vi "VolumeScan.vi"() -> ()   [LabVIEW 2015]
panel:
  out "Image":T1(plugin-control)
  out "Status":string
  in  "Capture":bool
  in  "Tab Control":T2(tab)
  in  "Frames per position":u32
  in  "Camera settings":bool
  out "Status":bool
  out "Temperature":dbl
  in  "Camera identity":u16(ring) items=["Andor Ixon", "Dummy", "Manual", "PCO Edge", "PointGrey Grasshopper"]
  in  "Exposure (s)":dbl=0.1
  in  "Volume Wizard":bool
  in  "Imaging Locations":dbl[][](array[numeric])
  in  "XYZ Position":dbl[](array[numeric])
  in  "Save":T3(ring)
  in  "Path":path=path "G:/"
  in  "File Prefix":string="Map"
  in  "Stage VISA":refnum<visa-resource-name>="COM5"
  in  "remote controlled":bool
  in  "closed loop controlled":bool
  in  "VISA resource name":refnum<visa-resource-name>="COM4"
  in  "Shut Down":bool
  # "Piezo"
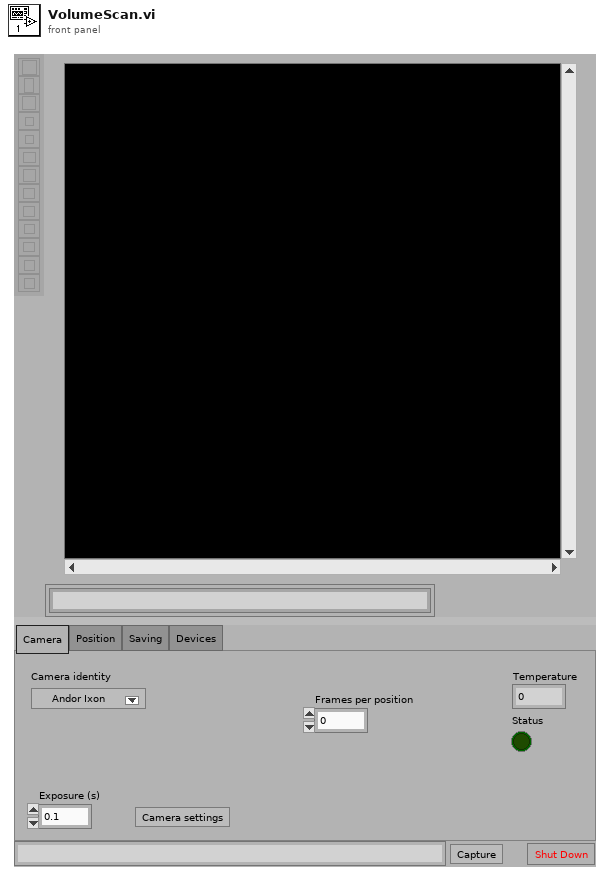
[diagram p1: front panel]
types:
  T1 = typedef "IMAQ Image.ctl" = refnum<image>
  T2 = enum32{"Camera", "Position", "Saving", "Devices"}
  T3 = enum16{"Don't save", "Save U16", "Save PNG", "Save TIFF"}
  T4 = enum16{"Initialize", "Shut down", "Set capture mode", "Set exposure", "Trigger and read", "Get status", "Other settings"}
  T5 = typedef "Image Type" = u32
  T6 = enum16{"Initialize", "Close", "Move Absolute", "Get Position", "Move Relative", "Set Acceleration", "Get Acceleration", "Set Speed", "Get Speed", "Limit Switch Status", "Motor Status", "Stop (controlled)", "Stop (instant)"}
  T7 = enum16{"Initialize", "Close", "Set position", "Get position", "Closed loop on", "Closed loop off", "Remote control on", "Remote control off"}
  T8 = cluster{"System OK?":bool, "Current exposure":dbl, "Temperature":dbl, "ROI":cluster{"X":u32, "X2":u32, "Y":u32, "Y2":u32}, "Binning":cluster{"X":u32, "Y":u32}}
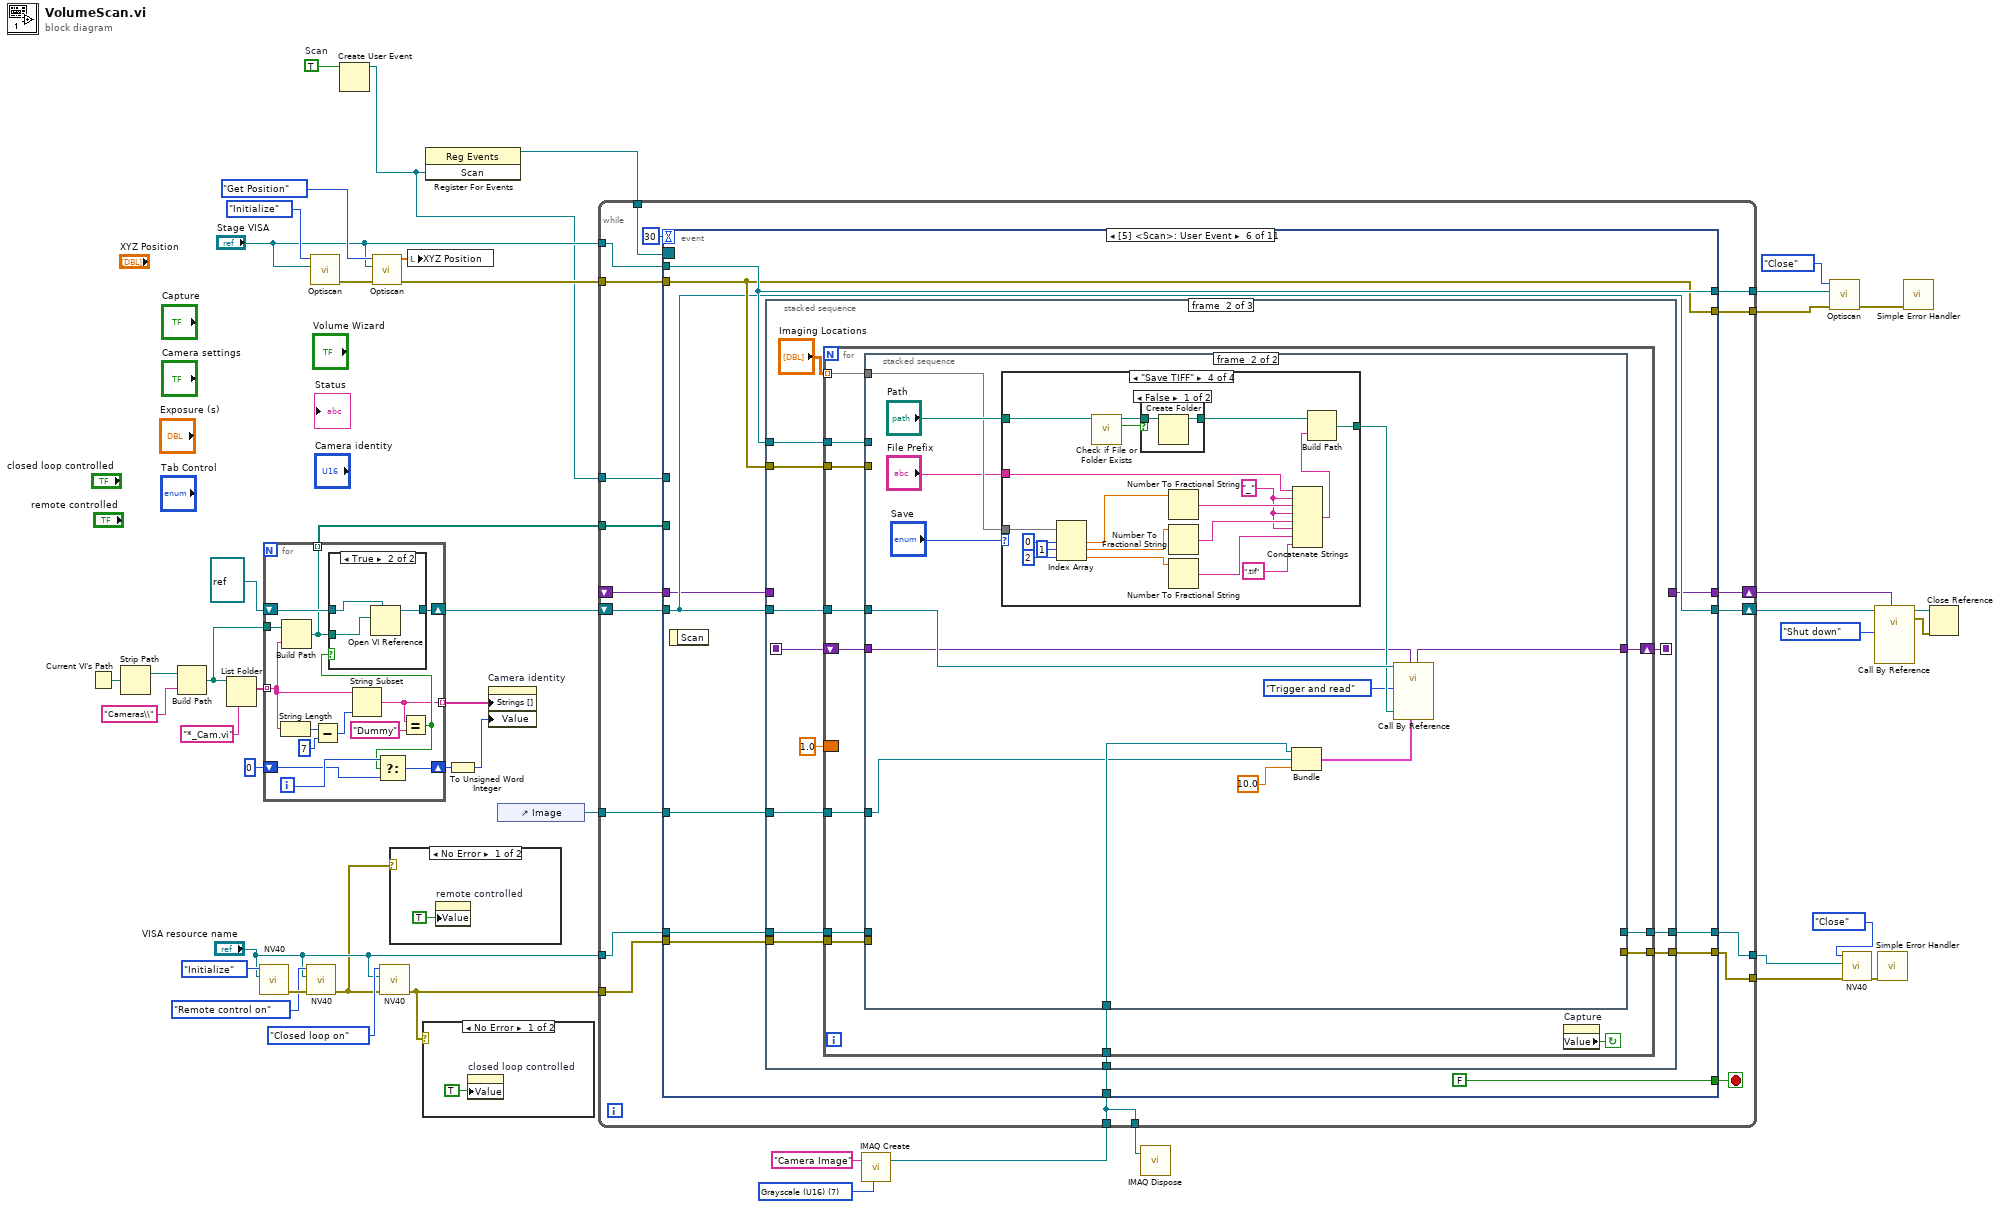
[diagram p0: block diagram]
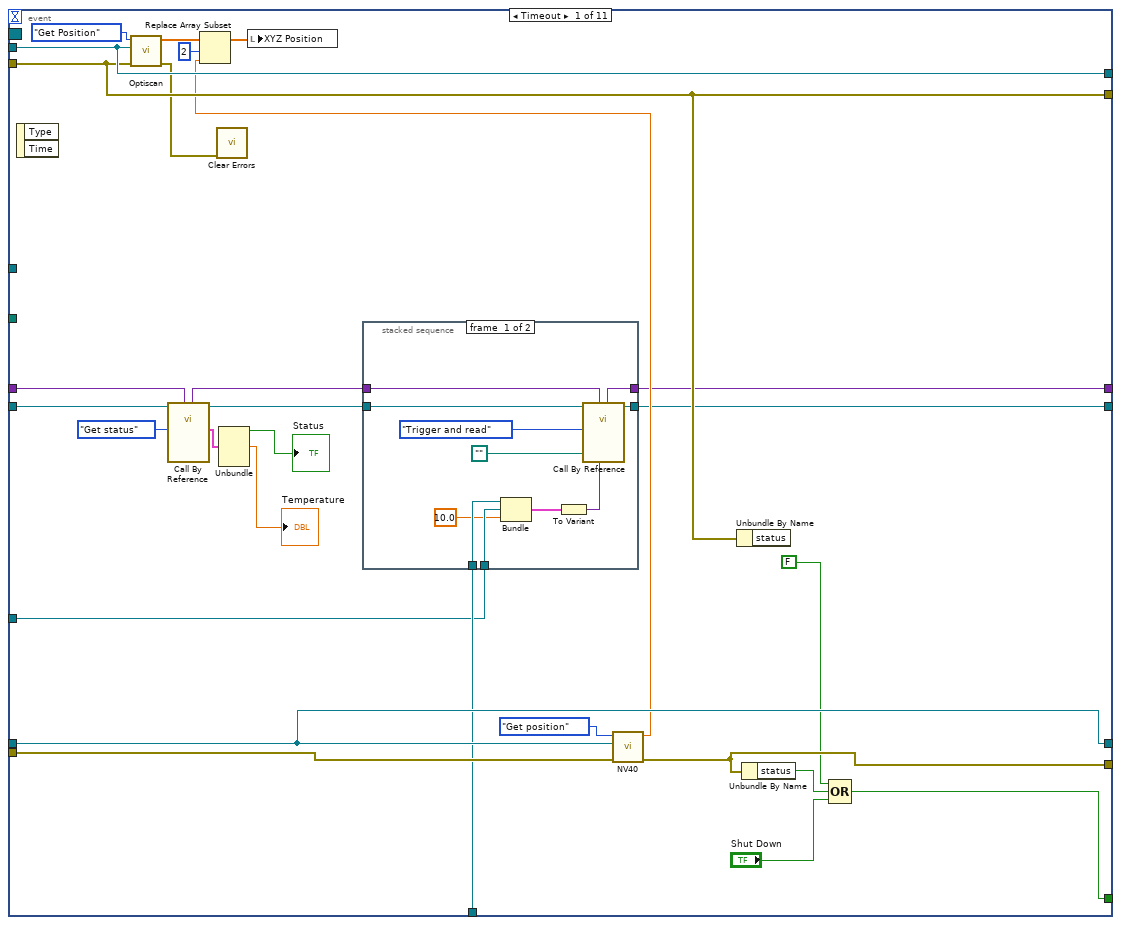
[diagram p5: hidden frame]
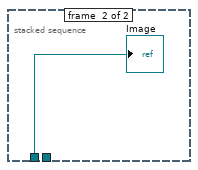
[diagram p6: hidden frame]
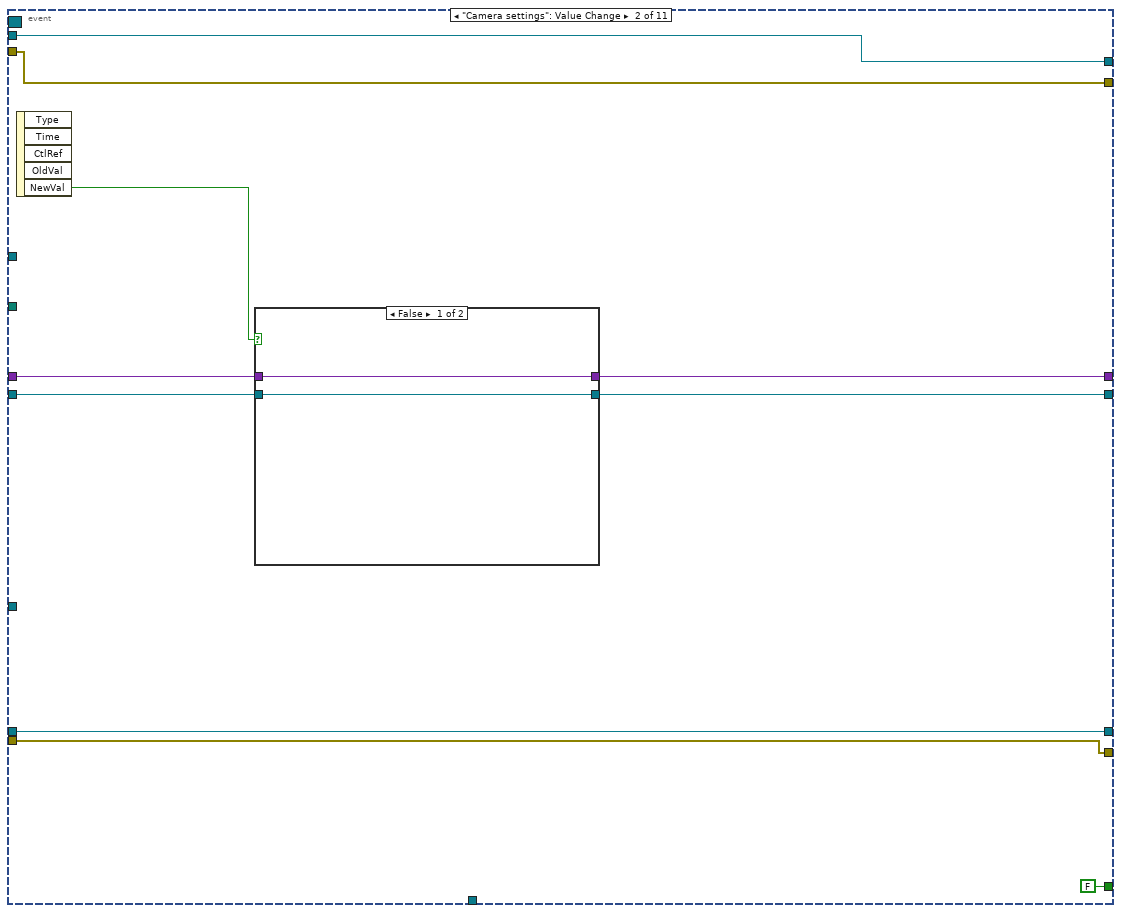
[diagram p7: hidden frame]
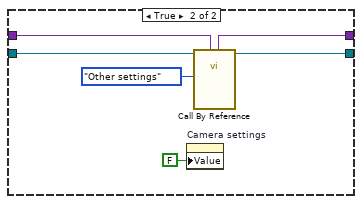
[diagram p8: hidden frame]
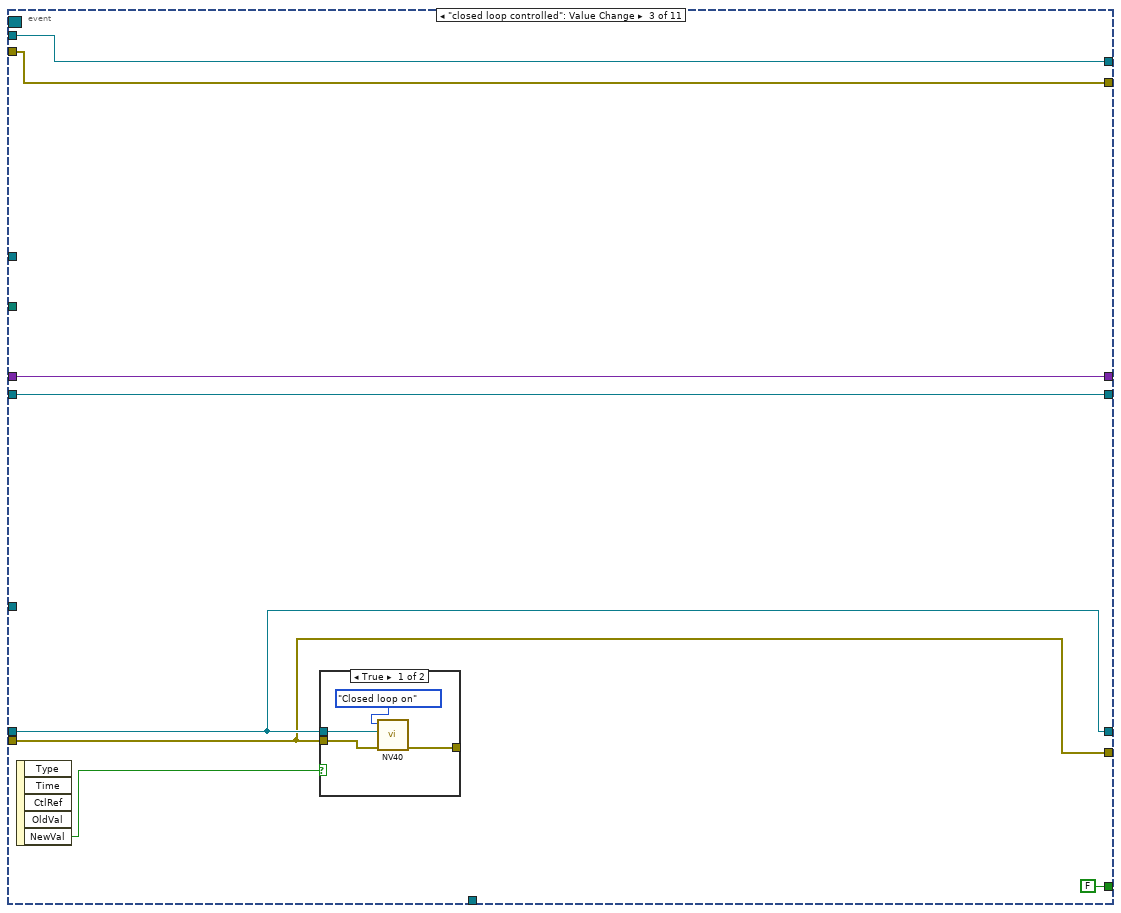
[diagram p9: hidden frame]
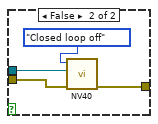
[diagram p10: hidden frame]
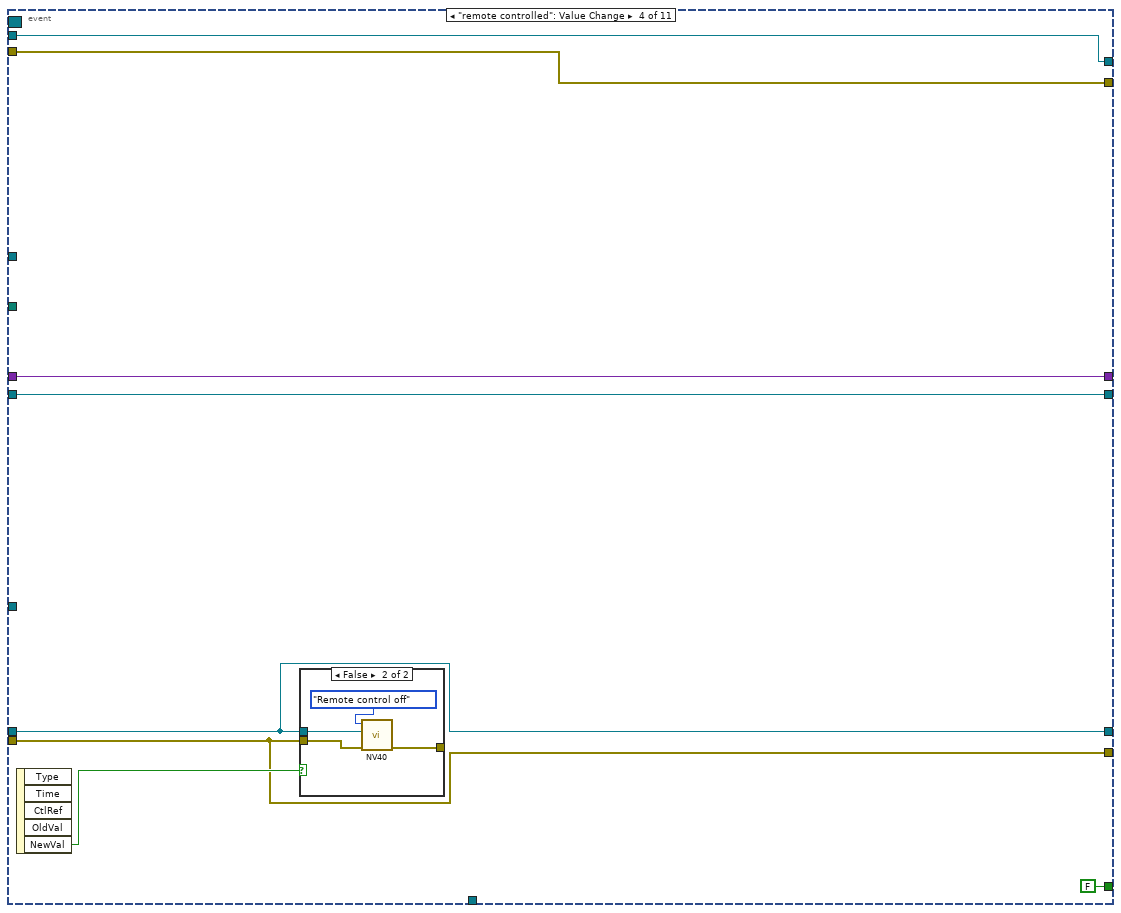
[diagram p11: hidden frame]
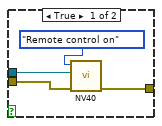
[diagram p12: hidden frame]
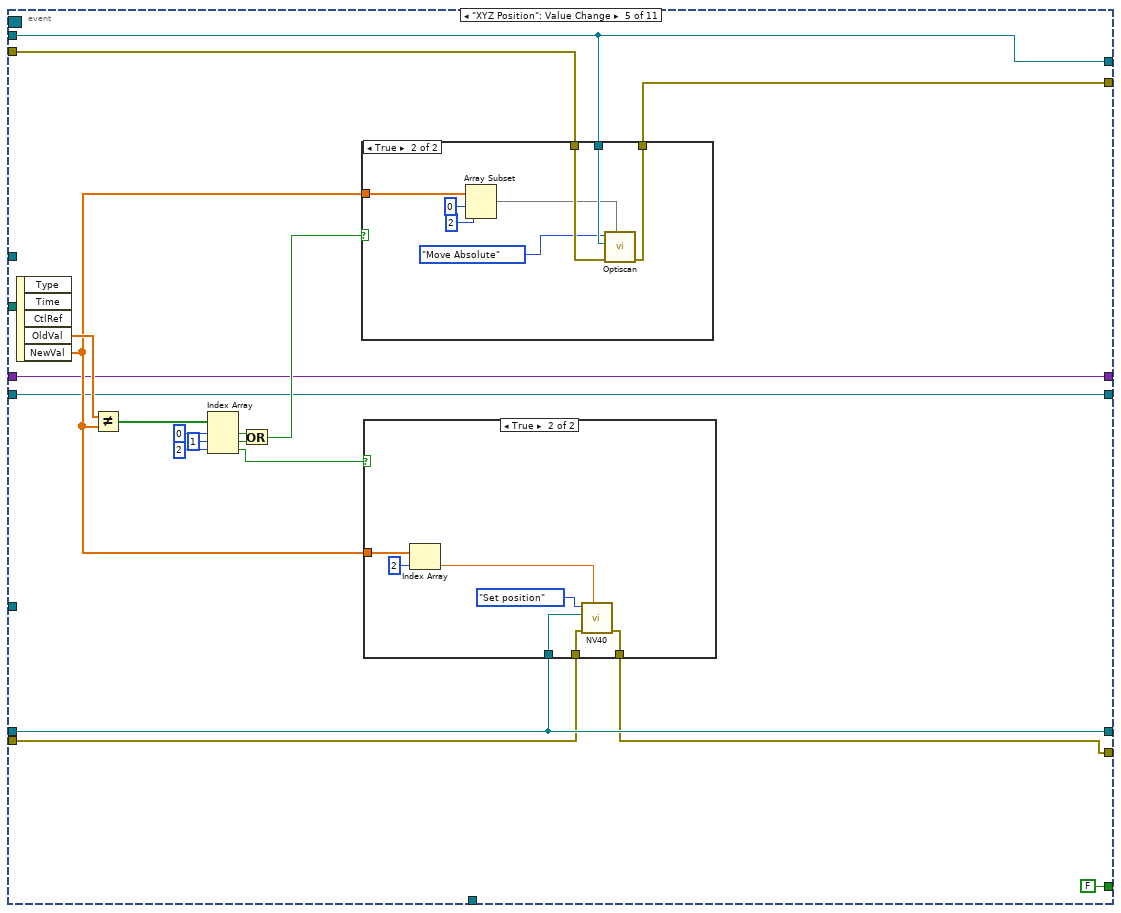
[diagram p13: hidden frame]
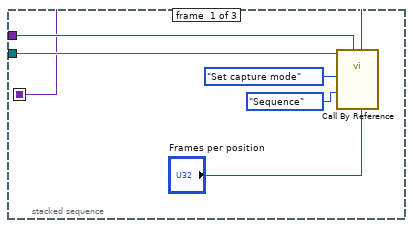
[diagram p16: hidden frame]
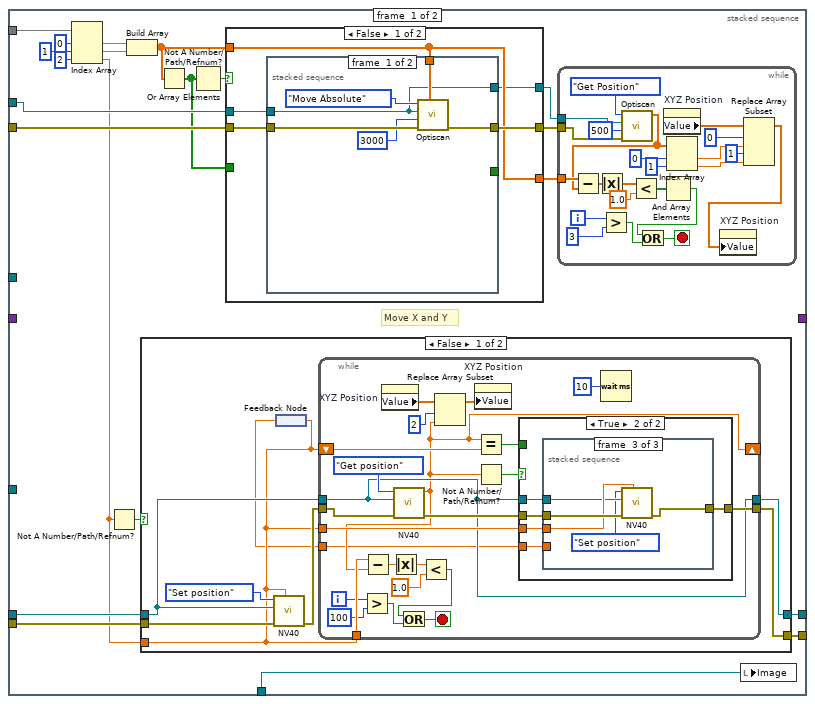
[diagram p17: hidden frame]
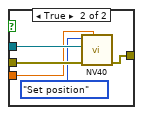
[diagram p19: hidden frame]
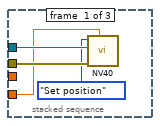
[diagram p20: hidden frame]
diagram:
  w6 = T5 7 items=["Grayscale (U8)", "Grayscale (I16)", "Grayscale (SGL)", "Complex (CSG)", "RGB (U32)", "HSL (U32)", "RGB (U64)", "Grayscale (U16)"] ("Image Type")
  w26 = TRUE  # Scan
  n1 = Current VI's Path() -> (path=w23:path)
  n2 = Strip Path(path=w23) -> (stripped path=w22:path)  [unwired: 1 out]
  n3 = Build Path(base path=w22, name or relative path="Cameras\\") -> (appended path=w15:path)
  n4 = List Folder(path=w15, pattern="*_Cam.vi") -> (filenames=w19:string[])  [unwired: 2 in, 3 out]
  n5 = call "NV40.vi"("VISA resource name"="VISA resource name", "Command"=T7."Initialize") -> ("error out"=w46:errorcluster)  [unwired: 5 in, 1 out]
  n6 = for {
    tunnel: w19 -> [w48] mode=indexing
    tunnel: [w50] -> w18 mode=indexing
    shift-right: [w59] -> w16
    shift-left: 0 -> [w58]
    tunnel: w15 -> [w54]
    shift-right: [w56] -> w14
    shift-left: refnum<vi> refnum ("type specifier VI Refnum (for type only)") -> [w55]
    tunnel: [w53] -> w12 mode=indexing
    i -> [w60]
    n7 = String Length(string=w48) -> (length=w52:i32)
    n8 = Build Path(base path=w54, name or relative path=w48) -> (appended path=w53:path)
    n9 = Subtract(x=w52, y=7) -> (x-y=w49:i32)
    n10 = String Subset(string=w48, length (rest)=w49) -> (substring=w50:string)  [unwired: 1 in]
    n11 = Equal?(x=w50, y="Dummy") -> (x = y?=w57:bool)
    n12 = case shown="True" w57 {
      tunnel: [w62 w65] -> w56
      tunnel: w55 -> [w62 w63]
      tunnel: w53 -> [_ w64]
      frame False {
      }
      frame True {
        n13 = Open VI Reference(type specifier VI Refnum (for type only)=w63, vi path=w64) -> (vi reference=w65:refnum<vi>)  [unwired: 4 in, 1 out]
      }
    }
    n14 = Select(t=w60, s=w57, f=w58) -> (s? t:f=w59:i32)
  }
  n15 = call "NV40.vi"("error in (no error)"=w46, "VISA resource name"="VISA resource name", "Command"=T7."Remote control on") -> ("error out"=w27:errorcluster)  [unwired: 4 in, 1 out]
  n16 = call "Optiscan.vi"("VISA resource name"="Stage VISA", "Command"=T6."Initialize") -> ("error out"=w37:errorcluster)  [unwired: 4 in, 2 out]
  n17 = Create User Event(user event datatype=w26) -> (user event=w24:refnum<user-event>)  [unwired: 1 in, 1 out]
  n18 = call "Optiscan.vi"("error in (no error)"=w37, "VISA resource name"="Stage VISA", "Command"=T6."Get Position") -> ("error out"=w36:errorcluster, "Parameter out"=w35:dbl[])  [unwired: 3 in, 1 out]
  n19 = call "NV40.vi"("error in (no error)"=w27, "VISA resource name"="VISA resource name", "Command"=T7."Closed loop on") -> ("error out"=w28:errorcluster)  [unwired: 4 in, 1 out]
  n20 = case shown="No Error" w27 {
    frame No Error {
      n21 = property on="remote controlled" class="Bool (strict)"("Value"=TRUE ("closed loop controlled")) -> ()  [unwired: 2 in, 2 out]
    }
    frame Error {
    }
  }
  n22 = local write "XYZ Position"(w35) -> ()
  n23 = case shown="No Error" w28 {
    frame No Error {
      n24 = property on="closed loop controlled" class="Bool (strict)"("Value"=TRUE ("closed loop controlled")) -> ()  [unwired: 2 in, 2 out]
    }
    frame Error {
    }
  }
  n25 = register-events(w24) -> (reference out=w25:refnum<event-registration>)  [unwired: 2 in, 1 out]
  n26 = To Unsigned Word Integer(number=w16) -> (unsigned 16bit integer=w3:u16)
  n27 = property on="Camera identity" class="Ring (strict)"("Strings []"=w18, "Value"=w3) -> ()  [unwired: 2 in, 2 out]
  n28 = control-ref of="Image"() -> (w1:refnum<vi>)
  n29 = call "IMAQ Create"("Image Name"="Camera Image", "Image Type"=w6) -> ("New Image"=w7:T1)  [unwired: 3 in, 1 out]
  n30 = while {
    tunnel: "VISA resource name" -> [w82]
    tunnel: w28 -> [w81]
    tunnel: [w84] -> w41
    tunnel: [w85] -> w42
    tunnel: w36 -> [w80]
    tunnel: "Stage VISA" -> [w79]
    tunnel: [w78] -> w32
    tunnel: [w77] -> w33
    tunnel: w25 -> [w76]
    tunnel: w24 -> [w75]
    shift-right: [w74] -> w9
    shift-left: w14 -> [w73]
    tunnel: w12 -> [w72]
    tunnel: w7 -> [w71]
    tunnel: [w71] -> w5
    shift-right: [w70] -> w2
    shift-left: _ -> [w69]
    tunnel: w1 -> [w68]
    stop <- w83 stop-if-true
    n31 = event shown="[5] <Scan>: User Event" {
      selector: w76 -> [_ _ _ _ _ _ _ _ _ _ _]
      dyn-events: _ -> [_ _ _ _ _ _ _ _ _ _ _]
      timeout: 30 -> [_ _ _ _ _ _ _ _ _ _ _]
      tunnel: [w109 w133 w151 w167 w182 w222 w486 w497 w510 w536 w553] -> w85
      tunnel: [w110 w132 w150 w166 w180 w221 w485 w496 w509 w535 w552] -> w84
      tunnel: [w112 FALSE FALSE FALSE FALSE FALSE FALSE FALSE FALSE FALSE FALSE] -> w83
      tunnel: w82 -> [w109 w133 w151 w167 w182 w224 w486 w497 w510 w536 w553]
      tunnel: w81 -> [w105 w132 w150 w166 w181 w223 w485 w496 w509 w535 w552]
      tunnel: w80 -> [w103 w135 w147 w164 w194 w218 w487 w498 w511 w532 w549]
      tunnel: w79 -> [w106 w136 w148 w165 w195 w219 w488 w499 w512 w533 w550]
      tunnel: [w103 w135 w147 w164 w193 w218 w487 w498 w511 w532 w549] -> w78
      tunnel: [w106 w136 w148 w165 w195 w219 w488 w499 w512 w533 w550] -> w77
      tunnel: w75 -> [_ _ _ _ _ _ w489 _ _ _ _]
      tunnel: [w95 w130 w146 w162 w178 w217 w483 w494 w507 w523 w546] -> w74
      tunnel: w73 -> [w100 w134 w146 w162 w178 w217 w483 w494 w507 w531 w548]
      tunnel: w72 -> [_ _ _ _ _ _ _ _ _ w540 _]
      tunnel: w71 -> [w88 _ _ _ _ w216 _ _ _ _ _]
      tunnel: [w91 w128 w145 w161 w177 w214 w482 w493 w506 w514 w541] -> w70
      tunnel: w69 -> [w93 w127 w145 w161 w177 w215 w482 w493 w506 w516 w542]
      tunnel: w68 -> [w87 _ _ _ _ w213 _ _ _ _ _]
      event Timeout {
        n32 = event-data() -> ()  [unwired: 1 in, 2 out]
        n33 = call "Optiscan.vi"("error in (no error)"=w103, "VISA resource name"=w106, "Command"=T6."Get Position") -> ("error out"=w89:errorcluster, "Parameter out"=w107:dbl[])  [unwired: 3 in, 1 out]
        n34 = call-by-ref "?"(reference=w100, "Camera-specific in"=w93, "Operation"=T4."Get status") -> (reference out=w99:refnum<vi>, "Status"=w98:T8, "Camera-specific out"=w92:variant)  [unwired: 9 in, 1 out]
        n35 = call <vilib>:"Clear Errors.vi"("error in (no error)"=w89) -> ()  [unwired: 5 in, 2 out]
        n36 = Unbundle(w98) -> ("System OK?"=→"Status":bool, "Temperature"=→"Temperature":dbl)  [unwired: 3 out]
        n37 = stacked-sequence {
          tunnel: w99 -> [w125 _]
          tunnel: [w124 _] -> w95
          tunnel: w92 -> [w121 _]
          tunnel: [w120 _] -> w91
          tunnel: w88 -> [w119 w126]
          tunnel: w87 -> [w117 _]
          frame #0 {
            n38 = Bundle("New Image"=w119, "Image"=w117, 10.0) -> (w118:cluster{"New Image":T1, "Image":refnum<vi>, dbl})  [unwired: 1 in]
            n39 = To Variant(anything=w118) -> (Variant=w116:variant)
            n40 = call-by-ref "?"(reference=w125, "Image in"=w116, "Camera-specific in"=w121, "Save path"=path "", "Operation"=T4."Trigger and read") -> (reference out=w124:refnum<vi>, "Camera-specific out"=w120:variant)  [unwired: 7 in, 2 out]
          }
          frame #1 {
            "Image" <- w126
          }
        }
        n41 = call "NV40.vi"("error in (no error)"=w105, "VISA resource name"=w109, "Command"=T7."Get position") -> ("error out"=w110:errorcluster, "Position out"=w102:dbl)  [unwired: 4 in]
        n42 = Replace Array Subset(array=w107, new element=w102, index=2) -> (w104:dbl[])
        n43 = local write "XYZ Position"(w104) -> ()
        n44 = Unbundle By Name(w103) -> ()  [unwired: 1 out]
        n45 = Unbundle By Name(w110) -> ("status"=w113:bool)
        n46 = Compound Arithmetic op=OR(FALSE ("value"), w113, "Shut Down") -> (w112:bool)
      }
      event "Camera settings": Value Change {
        n47 = event-data() -> ("NewVal"=w129:bool)  [unwired: 1 in, 4 out]
        n48 = case shown="False" w129 {
          tunnel: w134 -> [w138 w144]
          tunnel: [w138 w143] -> w130
          tunnel: [w137 w140] -> w128
          tunnel: w127 -> [w137 w139]
          frame False {
          }
          frame True {
            n49 = property on="Camera settings" class="Bool (strict)"("Value"=FALSE ("Camera settings")) -> ()  [unwired: 2 in, 2 out]
            n50 = call-by-ref "?"(reference=w144, "Camera-specific in"=w139, "Operation"=T4."Other settings") -> (reference out=w143:refnum<vi>, "Camera-specific out"=w140:variant)  [unwired: 9 in, 2 out]
          }
        }
      }
      event "closed loop controlled": Value Change {
        n51 = event-data() -> ("NewVal"=w152:bool)  [unwired: 1 in, 4 out]
        n52 = case shown="True" w152 {
          tunnel: w150 -> [w156 w160]
          tunnel: w151 -> [w155 w159]
          tunnel: [w153 w157] -> _
          frame True {
            n53 = call "NV40.vi"("error in (no error)"=w156, "VISA resource name"=w155, "Command"=T7."Closed loop on") -> ("error out"=w153:errorcluster)  [unwired: 4 in, 1 out]
          }
          frame False {
            n54 = call "NV40.vi"("error in (no error)"=w160, "VISA resource name"=w159, "Command"=T7."Closed loop off") -> ("error out"=w157:errorcluster)  [unwired: 4 in, 1 out]
          }
        }
      }
      event "remote controlled": Value Change {
        n55 = event-data() -> ("NewVal"=w168:bool)  [unwired: 1 in, 4 out]
        n56 = case shown="False" w168 {
          tunnel: w166 -> [w172 w176]
          tunnel: w167 -> [w171 w175]
          tunnel: [w169 w173] -> _
          frame True {
            n57 = call "NV40.vi"("error in (no error)"=w172, "VISA resource name"=w171, "Command"=T7."Remote control on") -> ("error out"=w169:errorcluster)  [unwired: 4 in, 1 out]
          }
          frame False {
            n58 = call "NV40.vi"("error in (no error)"=w176, "VISA resource name"=w175, "Command"=T7."Remote control off") -> ("error out"=w173:errorcluster)  [unwired: 4 in, 1 out]
          }
        }
      }
      event "XYZ Position": Value Change {
        n59 = event-data() -> ("OldVal"=w191:dbl[], "NewVal"=w179:dbl[])  [unwired: 1 in, 3 out]
        n60 = Not Equal?(x=w191, y=w179) -> (x != y?=w190:bool[])
        n61 = Index Array(array=w190, index #1=0 ("index"), index #2=1 ("index"), index #3=2 ("index")) -> (element #1=w186:bool, element #2=w185:bool, element #3=w183:bool)
        n62 = Or(x=w186, y=w185) -> (x .or. y?=w184:bool)
        n63 = case shown="True" w184 {
          tunnel: w195 -> [_ w212]
          tunnel: w194 -> [w204 w211]
          tunnel: [w204 w210] -> w193
          tunnel: w179 -> [_ w208]
          frame False {
          }
          frame True {
            n64 = Array Subset(array=w208, index=0, length=2) -> (w205:dbl[])
            n65 = call "Optiscan.vi"("Parameter in"=w205, "error in (no error)"=w211, "VISA resource name"=w212, "Command"=T6."Move Absolute") -> ("error out"=w210:errorcluster)  [unwired: 2 in, 2 out]
          }
        }
        n66 = case shown="True" w183 {
          tunnel: w182 -> [_ w202]
          tunnel: w181 -> [w196 w201]
          tunnel: [w196 w200] -> w180
          tunnel: w179 -> [_ w199]
          frame False {
          }
          frame True {
            n67 = Index Array(array=w199, index=2) -> (element=w197:dbl)
            n68 = call "NV40.vi"("Position"=w197, "error in (no error)"=w201, "VISA resource name"=w202, "Command"=T7."Set position") -> ("error out"=w200:errorcluster)  [unwired: 3 in, 1 out]
          }
        }
      }
      event User Event {
        n69 = event-data() -> ()  [unwired: 1 in, 1 out]
        n70 = stacked-sequence {
          seq-local: [w226 _ _] -> [_ w234 _]
          seq-local: [_ w233 _] -> [_ _ w477]
          tunnel: w224 -> [_ w243 _]
          tunnel: w223 -> [_ w242 _]
          tunnel: [_ w241 _] -> w222
          tunnel: [_ w240 _] -> w221
          tunnel: w219 -> [_ w238 _]
          tunnel: w218 -> [_ w237 _]
          tunnel: w217 -> [w230 w236 w479]
          tunnel: w216 -> [_ w235 _]
          tunnel: w215 -> [w227 _ _]
          tunnel: [_ _ w476] -> w214
          tunnel: w213 -> [_ w231 _]
          frame #0 {
            n71 = call-by-ref "?"(reference=w230, "Frames in sequence"="Frames per position", "Camera-specific in"=w227, "Capture mode"=enum16{"Single frame", "Sequence"}."Sequence", "Operation"=T4."Set capture mode") -> ("Camera-specific out"=w226:variant)  [unwired: 7 in, 3 out]
          }
          frame #1 {
            n72 = for {
              tunnel: w243 -> [w256]
              tunnel: w242 -> [w255]
              tunnel: [w254] -> w241
              tunnel: [w253] -> w240
              tunnel: "Imaging Locations" -> [w252] mode=indexing
              tunnel: w237 -> [w251]
              tunnel: w238 -> [w250]
              tunnel: w236 -> [w248]
              tunnel: w235 -> [w247]
              shift-right: [w245] -> w233
              shift-left: w234 -> [w246]
              border: 1.0 ("Numeric") -> [_]
              tunnel: w231 -> [w244]
              stop <- w249 continue-if-true
              n73 = stacked-sequence {
                tunnel: w256 -> [w274 _]
                tunnel: w255 -> [w275 _]
                tunnel: [w277 _] -> w254
                tunnel: [w276 _] -> w253
                tunnel: w252 -> [w273 w407]
                tunnel: w251 -> [w266 _]
                tunnel: w250 -> [w267 _]
                tunnel: w248 -> [_ w404]
                tunnel: w247 -> [w257 w399]
                tunnel: w246 -> [_ w401]
                tunnel: [_ w400] -> w245
                tunnel: w244 -> [_ w397]
                frame #0 {
                  # "Move X and Y"
                  n74 = Index Array(array=w273, index #1=0 ("index"), index #2=1 ("index"), index #3=2 ("index")) -> (element #1=w269:dbl, element #2=w268:dbl, element #3=w262:dbl)
                  n75 = Not A Number/Path/Refnum?(number/path/refnum=w262) -> (NaN/Path/Refnum?=w261:bool)
                  n76 = Build Array(w269, w268) -> (w263:dbl[])
                  n77 = case shown="False" w261 {
                    tunnel: [w308 w360] -> w277
                    tunnel: [w307 w359] -> w276
                    tunnel: w275 -> [w306 w359]
                    tunnel: w274 -> [w303 w360]
                    tunnel: w262 -> [w302 _]
                    frame False {
                      n78 = call "NV40.vi"("Position"=w302, "error in (no error)"=w306, "VISA resource name"=w303, "Command"=T7."Set position") -> ("error out"=w304:errorcluster)  [unwired: 3 in, 1 out]
                      n79 = feedback-in #1(w302) -> ()
                      n80 = feedback #1() -> (w301:dbl)
                      n81 = while {
                        tunnel: w303 -> [w313]
                        tunnel: w304 -> [w322]
                        tunnel: [w313] -> w308
                        tunnel: [w314] -> w307
                        tunnel: w302 -> [w332]
                        shift-right: [w311] -> _
                        shift-left: w302 -> [w312]
                        tunnel: w302 -> [w315]
                        tunnel: w301 -> [w309]
                        i -> [w328]
                        stop <- w326 stop-if-true
                        n82 = Greater?(x=w328, y=100) -> (0:w324:bool)
                        n83 = property on="XYZ Position" class="Arr (strict)"() -> ("Value"=w320:dbl[])  [unwired: 2 in, 2 out]
                        n84 = call "NV40.vi"("error in (no error)"=w322, "VISA resource name"=w313, "Command"=T7."Get position") -> ("error out"=w316:errorcluster, "Position out"=w311:dbl)  [unwired: 4 in]
                        n85 = Subtract(x=w332, y=w311) -> (x-y=w331:dbl)
                        n86 = Absolute Value(x=w331) -> (abs(x)=w330:dbl)
                        n87 = Less?(x=w330, y=1.0) -> (x < y?=w325:bool)
                        n88 = Or(x=w325, y=w324) -> (x .or. y?=w326:bool)
                        n89 = Replace Array Subset(array=w320, new element=w311, index=2) -> (w319:dbl[])
                        n90 = property on="XYZ Position" class="Arr (strict)"("Value"=w319) -> ()  [unwired: 2 in, 2 out]
                        n91 = Equal?(x=w311, y=w312) -> (x = y?=w317:bool)
                        n92 = Not A Number/Path/Refnum?(number/path/refnum=w311) -> (NaN/Path/Refnum?=w310:bool)
                        n93 = case shown="True" w310 {
                          tunnel: w317 -> [w337 _]
                          tunnel: w316 -> [w336 w348]
                          tunnel: w315 -> [w335 w347]
                          tunnel: [w334 w346] -> w314
                          tunnel: w313 -> [w333 w345]
                          tunnel: w309 -> [_ w344]
                          frame False {
                            n94 = case shown="False" w337 {
                              tunnel: w333 -> [_ w343]
                              tunnel: w336 -> [w338 w342]
                              tunnel: w335 -> [_ w341]
                              tunnel: [w338 w340] -> w334
                              frame False {
                              }
                              frame True {
                                n95 = call "NV40.vi"("Position"=w341, "error in (no error)"=w342, "VISA resource name"=w343, "Command"=T7."Set position") -> ("error out"=w340:errorcluster)  [unwired: 3 in, 1 out]
                              }
                            }
                          }
                          frame True {
                            n96 = stacked-sequence {
                              tunnel: w348 -> [w352 _ w358]
                              tunnel: w347 -> [_ _ w357]
                              tunnel: [_ _ w356] -> w346
                              tunnel: w345 -> [w351 _ w355]
                              tunnel: w344 -> [w349 _ _]
                              frame #0 {
                                n97 = call "NV40.vi"("Position"=w349, "error in (no error)"=w352, "VISA resource name"=w351, "Command"=T7."Set position") -> ()  [unwired: 3 in, 2 out]
                              }
                              frame #1 {
                                n98 = Wait (ms)(milliseconds to wait=u32 100) -> ()  [unwired: 1 out]
                              }
                              frame #2 {
                                n99 = call "NV40.vi"("Position"=w357, "error in (no error)"=w358, "VISA resource name"=w355, "Command"=T7."Set position") -> ("error out"=w356:errorcluster)  [unwired: 3 in, 1 out]
                              }
                            }
                          }
                        }
                        n100 = Wait (ms)(milliseconds to wait=u32 10) -> ()  [unwired: 1 out]
                      }
                    }
                    frame True {
                    }
                  }
                  n101 = Not A Number/Path/Refnum?(number/path/refnum=w263) -> (NaN/Path/Refnum?=w264:bool[])
                  n102 = Or Array Elements(Boolean array=w264) -> (logical OR=w265:bool)
                  n103 = case shown="False" w265 {
                    tunnel: w267 -> [w362 w382]
                    tunnel: w266 -> [w365 w390]
                    tunnel: w264 -> [_ w388]
                    tunnel: w263 -> [w363 w384]
                    tunnel: [w364 w383] -> w260
                    tunnel: [w361 w382] -> w259
                    tunnel: [w363 w381] -> w258
                    frame False {
                      n104 = stacked-sequence {
                        tunnel: w365 -> [w370 w373]
                        tunnel: [w369 _] -> w364
                        tunnel: w363 -> [w368 _]
                        tunnel: w362 -> [w367 w374]
                        tunnel: [w367 _] -> w361
                        tunnel: [_ w372] -> _
                        frame #0 {
                          n105 = call "Optiscan.vi"("Parameter in"=w368, "error in (no error)"=w370, "Timeout"=u32 3000, "VISA resource name"=w367, "Command"=T6."Move Absolute") -> ("error out"=w369:errorcluster)  [unwired: 1 in, 2 out]
                        }
                        frame #1 {
                          n106 = disable-structure shown="Disabled" {
                            disable-tunnel: w374 -> [w379 _]
                            disable-tunnel: w373 -> [w378 _]
                            disable-tunnel: [w377 _] -> w372
                            frame Disabled {
                              n107 = call "Optiscan.vi"("error in (no error)"=w378, "Timeout"=u32 500, "VISA resource name"=w379, "Command"=T6."Motor Status") -> ("Status out"=w377:bool[])  [unwired: 2 in, 2 out]
                            }
                            frame Enabled {
                            }
                          }
                        }
                      }
                    }
                    frame True {
                      n108 = call "Optiscan.vi"("error in (no error)"=w390, "VISA resource name"=w382, "Command"=T6."Get Position") -> ("error out"=w385:errorcluster, "Parameter out"=w387:dbl[])  [unwired: 3 in, 1 out]
                      n109 = for {
                        N: 2 -> [_]
                        tunnel: w388 -> [w395] mode=indexing
                        tunnel: w387 -> [w394] mode=indexing
                        tunnel: w384 -> [w393] mode=indexing
                        tunnel: [w392] -> w381 mode=indexing
                        n110 = Select(t=w394, s=w395, f=w393) -> (s? t:f=w392:dbl)
                      }
                      n111 = call "Optiscan.vi"("Parameter in"=w381, "error in (no error)"=w385, "Timeout"=u32 3000, "VISA resource name"=w382, "Command"=T6."Move Absolute") -> ("error out"=w383:errorcluster)  [unwired: 1 in, 2 out]
                    }
                  }
                  n112 = while {
                    tunnel: w259 -> [w291]
                    tunnel: w260 -> [w290]
                    tunnel: w258 -> [w289]
                    i -> [w297]
                    stop <- w295 stop-if-true
                    n113 = Greater?(x=w297, y=3) -> (0:w293:bool)
                    n114 = call "Optiscan.vi"("error in (no error)"=w290, "Timeout"=u32 500, "VISA resource name"=w291, "Command"=T6."Get Position") -> ("Parameter out"=w285:dbl[])  [unwired: 2 in, 2 out]
                    n115 = Subtract(x=w289, y=w285) -> (x-y=w300:dbl[])
                    n116 = Absolute Value(x=w300) -> (abs(x)=w299:dbl[])
                    n117 = Less?(x=w299, y=1.0) -> (x < y?=w294:bool[])
                    n118 = And Array Elements(Boolean array=w294) -> (logical AND=w288:bool)
                    n119 = Or(x=w288, y=w293) -> (x .or. y?=w295:bool)
                    n120 = property on="XYZ Position" class="Arr (strict)"() -> ("Value"=w287:dbl[])  [unwired: 2 in, 2 out]
                    n121 = Index Array(array=w285, index #1=0 ("index"), index #2=1 ("index")) -> (element #1=w281:dbl, element #2=w280:dbl)
                    n122 = Replace Array Subset(array=w287, new element #1=w281, index #1=0 ("index"), new element #2=w280, index #2=1 ("index")) -> (w286:dbl[])
                    n123 = property on="XYZ Position" class="Arr (strict)"("Value"=w286) -> ()  [unwired: 2 in, 2 out]
                  }
                  n124 = local write "Image"(w257) -> ()
                }
                frame #1 {
                  n125 = case shown="\"Save TIFF\"" "Save" {
                    tunnel: "Path" -> [_ w426 w448 w470]
                    tunnel: w407 -> [_ w421 w443 w465]
                    tunnel: "File Prefix" -> [_ w415 w437 w459]
                    tunnel: [path "" w410 w432 w454] -> w403
                    frame "Don't save", Default {
                    }
                    frame "Save U16" {
                      w414 = "_"
                      n126 = Index Array(array=w421, index #1=0 ("index"), index #2=1 ("index"), index #3=2 ("index")) -> (element #1=w413:dbl, element #2=w412:dbl, element #3=w411:dbl)
                      n127 = call <vilib>:"Check if File or Folder Exists.vi"("path"=w426) -> ("file or folder exists?"=w425:bool, "dup path"=w424:path)  [unwired: 8 in, 1 out]
                      n128 = case shown="False" w425 {
                        tunnel: w424 -> [w430 w431]
                        tunnel: [w429 w431] -> w423
                        frame False {
                          n129 = Create Folder(path (use dialog)=w430) -> (created path=w429:path)  [unwired: 2 in, 2 out]
                        }
                        frame True {
                        }
                      }
                      n130 = Number To Fractional String(number=w413) -> (F-format string=w428:string)  [unwired: 3 in]
                      n131 = Number To Fractional String(number=w412) -> (F-format string=w417:string)  [unwired: 3 in]
                      n132 = Number To Fractional String(number=w411) -> (F-format string=w416:string)  [unwired: 3 in]
                      n133 = Concatenate Strings(w415, w414, w428, w414, w417, w414, w416, ".U16") -> (w427:string)
                      n134 = Build Path(base path=w423, name or relative path=w427) -> (appended path=w410:path)
                    }
                    frame "Save PNG" {
                      w436 = "_"
                      n135 = Index Array(array=w443, index #1=0 ("index"), index #2=1 ("index"), index #3=2 ("index")) -> (element #1=w435:dbl, element #2=w434:dbl, element #3=w433:dbl)
                      n136 = call <vilib>:"Check if File or Folder Exists.vi"("path"=w448) -> ("file or folder exists?"=w447:bool, "dup path"=w446:path)  [unwired: 8 in, 1 out]
                      n137 = case shown="False" w447 {
                        tunnel: w446 -> [w452 w453]
                        tunnel: [w451 w453] -> w445
                        frame False {
                          n138 = Create Folder(path (use dialog)=w452) -> (created path=w451:path)  [unwired: 2 in, 2 out]
                        }
                        frame True {
                        }
                      }
                      n139 = Number To Fractional String(number=w435) -> (F-format string=w450:string)  [unwired: 3 in]
                      n140 = Number To Fractional String(number=w434) -> (F-format string=w439:string)  [unwired: 3 in]
                      n141 = Number To Fractional String(number=w433) -> (F-format string=w438:string)  [unwired: 3 in]
                      n142 = Concatenate Strings(w437, w436, w450, w436, w439, w436, w438, ".png") -> (w449:string)
                      n143 = Build Path(base path=w445, name or relative path=w449) -> (appended path=w432:path)
                    }
                    frame "Save TIFF" {
                      w458 = "_"
                      n144 = Index Array(array=w465, index #1=0 ("index"), index #2=1 ("index"), index #3=2 ("index")) -> (element #1=w457:dbl, element #2=w456:dbl, element #3=w455:dbl)
                      n145 = call <vilib>:"Check if File or Folder Exists.vi"("path"=w470) -> ("file or folder exists?"=w469:bool, "dup path"=w468:path)  [unwired: 8 in, 1 out]
                      n146 = case shown="False" w469 {
                        tunnel: w468 -> [w474 w475]
                        tunnel: [w473 w475] -> w467
                        frame False {
                          n147 = Create Folder(path (use dialog)=w474) -> (created path=w473:path)  [unwired: 2 in, 2 out]
                        }
                        frame True {
                        }
                      }
                      n148 = Number To Fractional String(number=w457) -> (F-format string=w472:string)  [unwired: 3 in]
                      n149 = Number To Fractional String(number=w456) -> (F-format string=w461:string)  [unwired: 3 in]
                      n150 = Number To Fractional String(number=w455) -> (F-format string=w460:string)  [unwired: 3 in]
                      n151 = Concatenate Strings(w459, w458, w472, w458, w461, w458, w460, ".tif") -> (w471:string)
                      n152 = Build Path(base path=w467, name or relative path=w471) -> (appended path=w454:path)
                    }
                  }
                  n153 = Bundle("New Image"=w399, "Image"=w397, 10.0) -> (w398:cluster{"New Image":T1, "Image":refnum<vi>, dbl})  [unwired: 1 in]
                  n154 = call-by-ref "?"(reference=w404, "Image in"=w398, "Camera-specific in"=w401, "Save path"=w403, "Operation"=T4."Trigger and read") -> ("Camera-specific out"=w400:variant)  [unwired: 7 in, 3 out]
                }
              }
              n155 = property on="Capture" class="Bool (strict)"() -> ("Value"=w249:bool)  [unwired: 2 in, 2 out]
            }
          }
          frame #2 {
            n156 = call-by-ref "?"(reference=w479, "Camera-specific in"=w477, "Capture mode"=enum16{"Single frame", "Sequence"}."Single frame", "Operation"=T4."Set capture mode") -> ("Camera-specific out"=w476:variant)  [unwired: 8 in, 3 out]
            n157 = property on="Capture" class="Bool (strict)"("Value"=FALSE ("Capture")) -> ()  [unwired: 2 in, 2 out]
          }
        }
      }
      event "Capture": Value Change {
        n158 = event-data() -> ("NewVal"=w490:bool)  [unwired: 1 in, 1 out]
        n159 = case shown="True" w490 {
          tunnel: w489 -> [_ w492]
          frame False {
          }
          frame True {
            n160 = Generate User Event(user event=w492, event data cluster=TRUE ("event data")) -> ()  [unwired: 2 in, 2 out]
          }
        }
      }
      event "Volume Wizard": Value Change {
        n161 = event-data() -> ("NewVal"=w500:bool)  [unwired: 1 in, 4 out]
        n162 = case shown="True" w500 {
          tunnel: w499 -> [_ w505]
          tunnel: w497 -> [_ w504]
          frame False {
          }
          frame True {
            n163 = property on="Imaging Locations" class="Arr (strict)"() -> ("Value"=w503:dbl[][])  [unwired: 2 in, 2 out]
            n164 = call "VolumeScanWizard.vi"("Piezo in"=w504, "XY in"=w505, "Coordinates in"=w503) -> ("Coordinates out"=w502:dbl[][])  [unwired: 8 in]
            n165 = property on="Imaging Locations" class="Arr (strict)"("Value"=w502) -> ()  [unwired: 2 in, 2 out]
            n166 = property on="Volume Wizard" class="Bool (strict)"("Value"=FALSE ("Volume Wizard")) -> ()  [unwired: 2 in, 2 out]
          }
        }
      }
      event "Tab Control": Value Change {
        n167 = event-data() -> ("NewVal"=w513:T2)  [unwired: 1 in, 4 out]
        n168 = case shown="\"Position\"" w513 {
          frame "Camera", Default {
          }
          frame "Position" {
          }
        }
      }
      event "Camera identity": Value Change {
        n169 = event-data() -> ("NewVal"=w539:u16)  [unwired: 1 in, 4 out]
        n170 = call <vilib>:"Set Busy.vi"() -> ("error out"=w521:errorcluster)  [unwired: 10 in, 1 out]
        n171 = call-by-ref "?"(reference=w531, error in=w521, "Camera-specific in"=w516, "Operation"=T4."Shut down") -> (reference out=w530:refnum<vi>, error out=w528:errorcluster)  [unwired: 8 in, 2 out]
        n172 = Close Reference(reference=w530, error in (no error)=w528) -> (error out=w529:errorcluster)
        n173 = Index Array(array=w540, index=w539) -> (element=w538:path)
        n174 = Open VI Reference(type specifier VI Refnum (for type only)=w530, vi path=w538, error in (no error)=w529) -> (vi reference=w537:refnum<vi>)  [unwired: 3 in, 1 out]
        n175 = property on="Exposure (s)" class="DigNum (strict)"() -> ("Value"=w526:dbl)  [unwired: 2 in, 2 out]
        n176 = call-by-ref "?"(reference=w537, "Exposure time (s)"=w526, "Operation"=T4."Initialize") -> (reference out=w527:refnum<vi>, "Status"=w525:T8, "Camera-specific out"=w515:variant)  [unwired: 9 in, 1 out]
        n177 = Unbundle By Name(w525) -> ("Current exposure"=w524:dbl)
        n178 = property on="Exposure (s)" class="DigNum (strict)"("Value"=w524) -> ()  [unwired: 2 in, 2 out]
        n179 = call-by-ref "?"(reference=w527, "Camera-specific in"=w515, "Capture mode"=enum16{"Single frame", "Sequence"}."Single frame", "Operation"=T4."Set capture mode") -> (reference out=w523:refnum<vi>, error out=w520:errorcluster, "Camera-specific out"=w514:variant)  [unwired: 8 in, 1 out]
        n180 = call <vilib>:"Unset Busy.vi"("error in (no error)"=w520) -> ()  [unwired: 10 in, 1 out]
      }
      event "Exposure (s)": Value Change {
        n181 = event-data() -> ("NewVal"=w547:dbl)  [unwired: 1 in, 4 out]
        n182 = call-by-ref "?"(reference=w548, "Camera-specific in"=w542, "Exposure time (s)"=w547, "Operation"=T4."Set exposure") -> (reference out=w546:refnum<vi>, "Status"=w545:T8, "Camera-specific out"=w541:variant)  [unwired: 8 in, 1 out]
        n183 = Unbundle By Name(w545) -> ("Current exposure"=w544:dbl)
        n184 = property on="Exposure (s)" class="DigNum (strict)"("Value"=w544) -> ()  [unwired: 2 in, 2 out]
      }
    }
  }
  n185 = call "IMAQ Dispose"("Image"=w5) -> ()  [unwired: 5 in, 1 out]
  n186 = call "Optiscan.vi"("error in (no error)"=w32, "VISA resource name"=w33, "Command"=T6."Close") -> ("error out"=w30:errorcluster)  [unwired: 3 in, 2 out]
  n187 = call "NV40.vi"("error in (no error)"=w41, "VISA resource name"=w42, "Command"=T7."Close") -> ("error out"=w43:errorcluster)  [unwired: 4 in, 1 out]
  n188 = call-by-ref "?"(reference=w9, "Camera-specific in"=w2, "Operation"=T4."Shut down") -> (reference out=w10:refnum<vi>, error out=w11:errorcluster)  [unwired: 9 in, 2 out]
  n189 = call <vilib>:"Simple Error Handler.vi"("error in (no error)"=w43) -> ()  [unwired: 4 in, 5 out]
  n190 = call <vilib>:"Simple Error Handler.vi"("error in (no error)"=w30) -> ()  [unwired: 4 in, 5 out]
  n191 = Close Reference(reference=w10, error in (no error)=w11) -> ()  [unwired: 1 out]
